vi "ObtainControlNames.vi"(8 "error in (no error)":errorcluster, 10 "AddedPrefix":string, 11 "ControlRefnumArray":refnum<vi>[](array[refnum])) -> (0 "error out":errorcluster, 3 "ControlNamesArray":string[](array[string]))   [LabVIEW 2016, in "M1M3SupportEUI_Views.lvlib"]
uses:
  M1M3SupportEUI_Views.lvlib
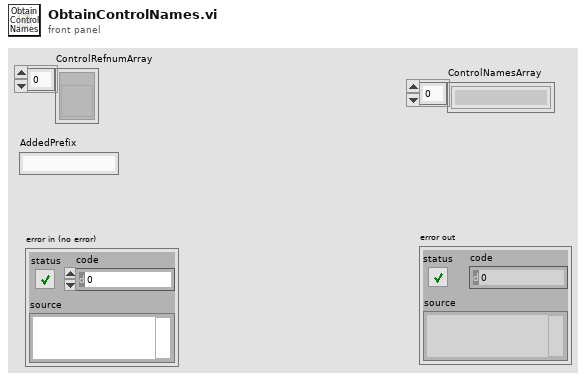
[diagram p1: front panel]
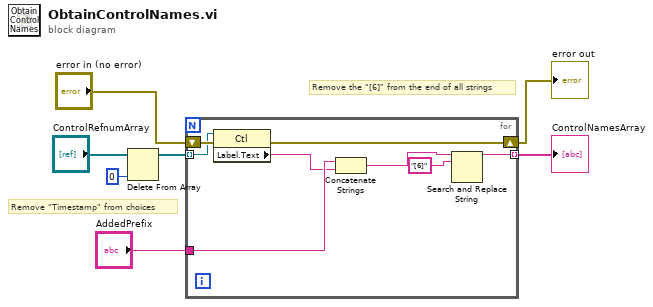
[diagram p0: block diagram]
diagram:
  # "Remove the \"[6]\" from the end of all strings"
  # "Remove \"Timestamp\" from choices"
  n1 = Delete From Array(array="ControlRefnumArray", index=0) -> (array with subset deleted=w7:refnum<vi>[])  [unwired: 1 in, 1 out]
  n2 = for {
    shift-right: [w14] -> w4
    shift-left: "error in (no error)" -> [w15]
    tunnel: w7 -> [w13] mode=indexing
    tunnel: [w11] -> w5 mode=indexing
    tunnel: "AddedPrefix" -> [w9]
    n3 = property class="Ctl"(reference=w13, error in=w15) -> (error out=w14:errorcluster, "Label.Text"=w8:string)  [unwired: 1 out]
    n4 = Concatenate Strings(w9, w8) -> (w10:string)
    n5 = Search and Replace String(input string=w10, search string="[6]") -> (result string=w11:string)  [unwired: 6 in, 3 out]
  }
  "ControlNamesArray" <- w5
  "error out" <- w4
